vi "Vision Processing.vi"(4 "error in (no error)":errorcluster, 7 "Image Size":T1=enum."320x240") -> ()   [LabVIEW 2018]
doc: "This VI runs in parallel to other tasks. It gets images from the camera, processes them for color or shape and use that information to affect robot behavior."
uses:
  <vilib>/Rock Robotics/WPI/Camera/WPI_CameraImageSize.ctl
  <vilib>/Rock Robotics/WPI/Camera/WPI_CameraWhite Balance Values.ctl
  <vilib>/Rock Robotics/WPI/Camera/WPI_CameraFrameRate.ctl
  Robot Global Data.vi
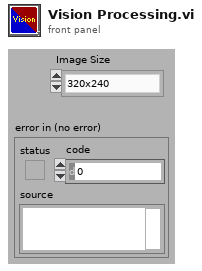
[diagram p1: front panel]
types:
  T1 = typedef "WPI_CameraImageSize.ctl" = enum16{"640x480", "320x240", "160x120", "Custom"}
  T2 = typedef "WPI_CameraFrameRate.ctl" = u32
  T3 = typedef "WPI_CameraWhite Balance Values.ctl" = enum16{"Auto", "Fixed indoor", "Fixed outdoor 1", "Fixed outdoor 2", "Fixed fluorescent 1", "Fixed fluorescent 2", "Hold current", "Custom"}
  T4 = typedef "Image Type" = u32
  T5 = typedef "WPI_CameraDevRef.ctl" = cluster{"Camera Address":string, "CameraStatus":errorcluster}
  T6 = typedef "IMAQ Image.ctl" = refnum<image>
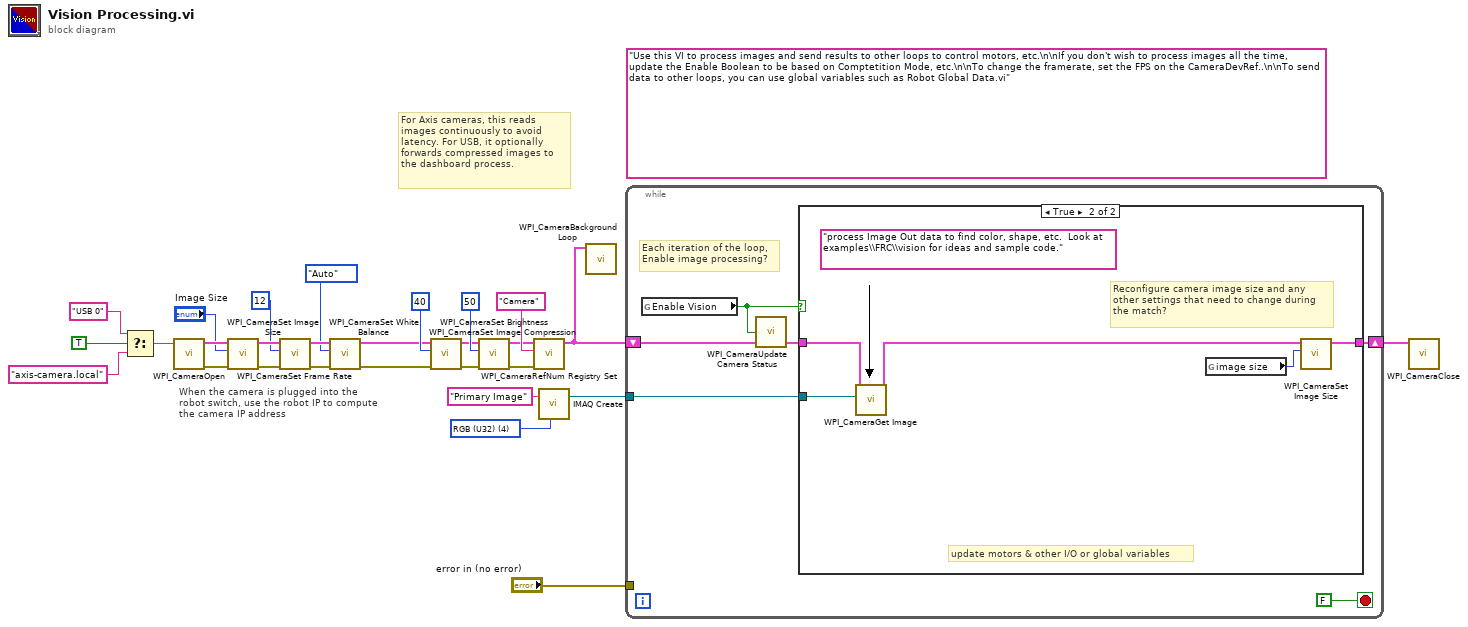
[diagram p0: block diagram]
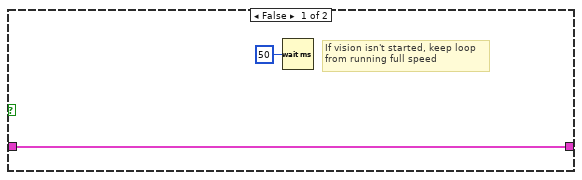
[diagram p2: hidden frame]
diagram:
  (unwired) "Use this VI to process images and send results to other loops to control motors, etc.\n\nIf you don't wish to process images all the time, update the Enable Boolean to be based on Comptetition Mode, etc.\n\nTo change the framerate, set the FPS on the CameraDevRef..\n\nTo send data to other loops, you can use global variables such as Robot Global Data.vi"
  w28 = T4 4 items=["Grayscale (U8)", "Grayscale (I16)", "Grayscale (SGL)", "Complex (CSG)", "RGB (U32)", "HSL (U32)", "RGB (U64)"] ("Image Type")
  # "When the camera is plugged into the\nrobot switch, use the robot IP to compute\nthe camera IP address"
  # "For Axis cameras, this reads\nimages continuously to avoid\nlatency. For USB, it optionally\nforwards compressed images to\nthe dashboard process."
  n1 = Select(t="USB 0" ("format string"), s=TRUE ("dot notation? (F)"), f="axis-camera.local" ("format string")) -> (s? t:f=w4:string)
  n2 = call <vilib>:"WPI_CameraOpen.vi"("Camera Address"=w4) -> ("error out"=w18:errorcluster, "CameraDevRef"=w19:T5)  [unwired: 1 in, 8 out]
  n3 = call <vilib>:"WPI_CameraSet Image Size.vi"("error in (no error)"=w18, "Image Size"="Image Size", "CameraDevRef"=w19) -> ("error out"=w17:errorcluster, "CameraDevRef Out"=w20:T5)  [unwired: 1 in, 6 out]
  n4 = call <vilib>:"WPI_CameraSet Frame Rate.vi"("error in (no error)"=w17, "Frame Rate (fps)"=T2 12, "CameraDevRef"=w20) -> ("error out"=w16:errorcluster, "CameraDevRef Out"=w21:T5)  [unwired: 7 out]
  n5 = call <vilib>:"WPI_CameraSet White Balance.vi"("error in (no error)"=w16, "White Balance"=WPI_CameraWhite_Balance_Values."Auto", "CameraDevRef"=w21) -> ("error out"=w1:errorcluster, "CameraDevRef Out"=w2:T5)  [unwired: 1 in, 6 out]
  n6 = call <vilib>:"WPI_CameraSet Image Compression.vi"("error in (no error)"=w1, "Compression"=40, "CameraDevRef"=w2) -> ("error out"=w15:errorcluster, "CameraDevRef Out"=w22:T5)  [unwired: 7 out]
  n7 = call <vilib>:"WPI_CameraSet Brightness.vi"("error in (no error)"=w15, "Brightness"=50, "CameraDevRef"=w22) -> ("error out"=w13:errorcluster, "CameraDevRef Out"=w14:T5)  [unwired: 1 in, 6 out]
  n8 = call <vilib>:"WPI_CameraRefNum Registry Set.vi"("error in (no error)"=w13, "refnum name"="Camera", "CameraDevRef"=w14) -> ("CameraDevRef"=w10:T5)  [unwired: 1 in, 7 out]
  n9 = call "IMAQ Create"("Image Name"="Primary Image", "Image Type"=w28) -> ("New Image"=w26:T6)  [unwired: 2 in, 2 out]
  n10 = call <vilib>:"WPI_CameraBackground Loop.vi"("CameraDevRef"=w10) -> ()  [unwired: 11 in]
  n11 = while {
    shift-right: [w33] -> w8
    shift-left: w10 -> [w31]
    tunnel: w26 -> [w32]
    tunnel: "error in (no error)" -> [_]
    stop <- FALSE stop-if-true
    # "Each iteration of the loop,\nEnable image processing?"
    n12 = global read "Robot Global Data.vi" "Enable Vision"() -> (w29:bool)
    n13 = call <vilib>:"WPI_CameraUpdate Camera Status.vi"("CameraDevRef In"=w31, "Enable Vision"=w29) -> ("CameraDevRef Out"=w30:T5)  [unwired: 3 in]
    n14 = case shown="True" w29 {
      tunnel: w32 -> [_ w40]
      tunnel: [w36 w41] -> w33
      tunnel: w30 -> [w36 w38]
      frame False {
        # "If vision isn't started, keep loop\nfrom running full speed"
        n15 = Wait (ms)(milliseconds to wait=u32 50) -> ()  [unwired: 1 out]
      }
      frame True {
        (unwired) "process Image Out data to find color, shape, etc.  Look at examples\\FRC\\vision for ideas and sample code."
        # "update motors & other I/O or global variables"
        # "Reconfigure camera image size and any\nother settings that need to change during\nthe match?"
        n16 = call <vilib>:"WPI_CameraGet Image.vi"("Image"=w40, "CameraDevRef"=w38) -> ("CameraDevRef Out"=w37:T5)  [unwired: 1 in, 8 out]
        n17 = global read "Robot Global Data.vi" "image size"() -> (w39:T1)
        n18 = call <vilib>:"WPI_CameraSet Image Size.vi"("Image Size"=w39, "CameraDevRef"=w37) -> ("CameraDevRef Out"=w41:T5)  [unwired: 2 in, 7 out]
      }
    }
  }
  n19 = call <vilib>:"WPI_CameraClose.vi"("CameraDevRef"=w8) -> ()  [unwired: 1 in, 10 out]
